vi "Add Three Inputs.vi"(2 "in 2":sgl, 6 "in 3":sgl, 10 "in 1":sgl) -> (5 "Numeric":sgl)   [LabVIEW 2014]
doc: "Simple add but with three inputs."
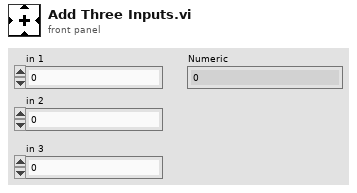
[diagram p1: front panel]
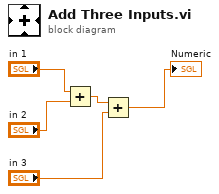
[diagram p0: block diagram]
diagram:
  n1 = Add(x="in 1", y="in 2") -> (x+y=w3:sgl)
  n2 = Add(x=w3, y="in 3") -> (x+y=→"Numeric":sgl)
